vi "Finish.vi"   [LabVIEW 2016]
doc: "This VI is called just before exiting. It is expected to close I/O refnum, save collected data, etc."
uses:
  <vilib>/Rock Robotics/WPI/Utilities/WPI_GetSetVariantRefNum.vi
types:
  T1 = typedef "WPI_MotorControlDeviceRef.ctl" = cluster{"DeviceStatus":errorcluster, "Type":T2, "PWM":cluster{"PWM Channel":T3, "DeadBand":T4}, "CAN":cluster{"Device Number":u8, "SetOutput VI Ref":variant, "GetOutput VI Ref":variant, "Enable VI Ref":variant, "Disable VI Ref":variant, "Data":variant}, "Invert":bool}
  T2 = typedef "WPI_MotorControlType.ctl" = enum16{"PWM", "CAN"}
  T3 = typedef "FPGA_DIOPWMChannel.ctl" = enum8{"PWM 0", "PWM 1", "PWM 2", "PWM 3", "PWM 4", "PWM 5", "PWM 6", "PWM 7", "PWM 8", "PWM 9", "PWM MXP 0", "PWM MXP 1", "PWM MXP 2", "PWM MXP 3", "PWM MXP 4", "PWM MXP 5", "PWM MXP 6", "PWM MXP 7", "PWM MXP 8", "PWM MXP 9", "Invalid"}
  T4 = typedef "WPI_PWMDeadband.ctl" = cluster{"Name":string, "maxPositivePwm":i32, "minPositivePwm":i32, "centerPwm":i32, "maxNegativePwm":i32, "minNegativePwm":i32, "angularRange":u16}
  T5 = typedef "WPI_RelayDevRef.ctl" = cluster{"DevStatus":errorcluster, "Relay Channel":T6, "Relay Direction":T7}
  T6 = typedef "FPGA_DIORelayChannel.ctl" = enum8{"Relay 0", "Relay 1", "Relay 2", "Relay 3", "Invalid"}
  T7 = typedef "WPI_RelayDirection.ctl" = enum16{"Both directions", "Forward only", "Reverse only"}
  T8 = typedef "WPI_JoystickDevRef.ctl" = cluster{"Device":T9}
  T9 = typedef "WPI_JoystickDeviceEnum.ctl" = enum16{"USB 0", "USB 1", "USB 2", "USB 3", "USB 4", "USB 5"}
  T10 = typedef "WPI_RobotDriveDevRef.ctl" = cluster{"DevStatus":errorcluster, "Motors[]":T1[], "Square Inputs":bool, "Max Output":dbl}
  T11 = typedef "WPI_SolenoidDevRef.ctl" = cluster{"DevStatus":errorcluster, "Pneumatics Control Module":u8, "Forward Solenoid Channel":T12, "Reverse Solenoid Channel":T12}
  T12 = typedef "WPI_SolenoidChannel.ctl" = enum8{"Solenoid 0", "Solenoid 1", "Solenoid 2", "Solenoid 3", "Solenoid 4", "Solenoid 5", "Solenoid 6", "Solenoid 7", "Invalid"}
  T13 = typedef "WPI_CompressorDevRef.ctl" = cluster{"DevStatus":errorcluster, "Pneumatics Control Module":u8}
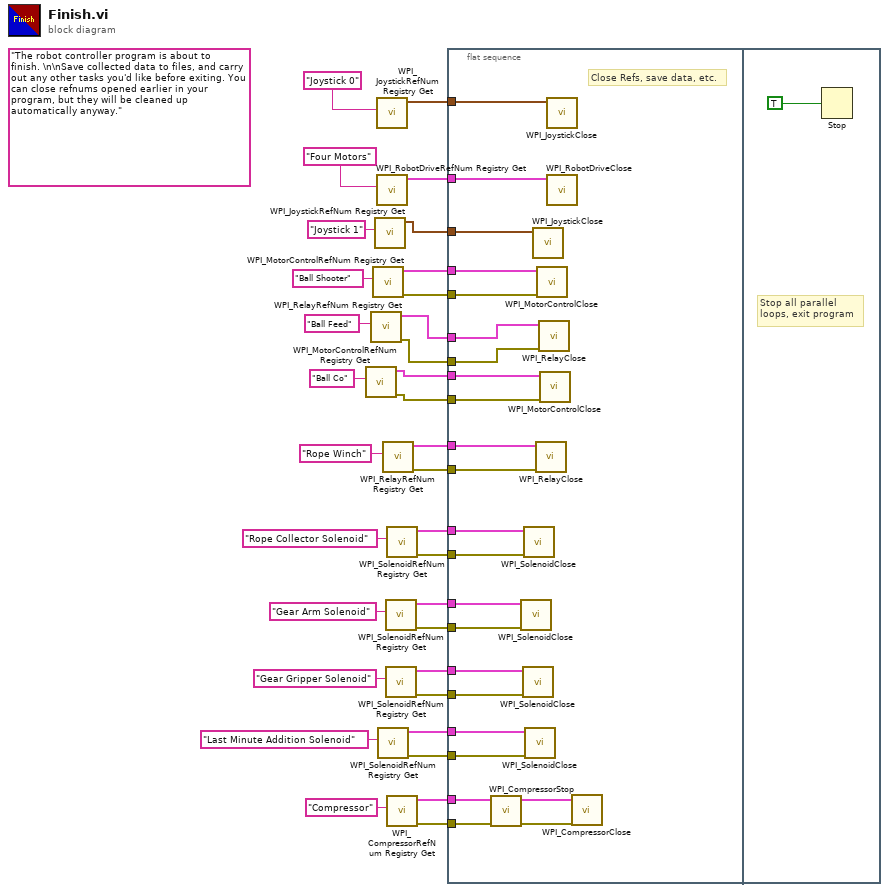
[diagram p0: block diagram]
diagram:
  (unwired) "The robot controller program is about to finish. \n\nSave collected data to files, and carry out any other tasks you'd like before exiting. You can close refnums opened earlier in your program, but they will be cleaned up automatically anyway."
  n1 = call <vilib>:"WPI_MotorControlRefNum Registry Get.vi"("refnum name"="Ball Co") -> ("error out"=w19:errorcluster, "MotorControlDevRef"=w20:T1)  [unwired: 9 in]
  n2 = call <vilib>:"WPI_RelayRefNum Registry Get.vi"("refnum name"="Ball Feed") -> ("error out"=w22:errorcluster, "RelayDevRef"=w23:T5)  [unwired: 9 in]
  n3 = call <vilib>:"WPI_MotorControlRefNum Registry Get.vi"("refnum name"="Ball Shooter") -> ("error out"=w25:errorcluster, "MotorControlDevRef"=w26:T1)  [unwired: 9 in]
  n4 = call <vilib>:"WPI_JoystickRefNum Registry Get.vi"("refnum name"="Joystick 1") -> ("JoystickDevRef"=w28:T8)  [unwired: 1 in, 9 out]
  n5 = call <vilib>:"WPI_JoystickRefNum Registry Get.vi"("refnum name"="Joystick 0") -> ("JoystickDevRef"=w30:T8)  [unwired: 1 in, 9 out]
  n6 = call <vilib>:"WPI_RobotDriveRefNum Registry Get.vi"("refnum name"="Four Motors") -> ("RobotDriveDevRef"=w31:T10)  [unwired: 1 in, 9 out]
  n7 = call <vilib>:"WPI_SolenoidRefNum Registry Get.vi"("refnum name"="Last Minute Addition Solenoid") -> ("error out"=w2:errorcluster, "SolenoidDevRef"=w3:T11)  [unwired: 9 in]
  n8 = call <vilib>:"WPI_RelayRefNum Registry Get.vi"("refnum name"="Rope Winch") -> ("error out"=w16:errorcluster, "RelayDevRef"=w17:T5)  [unwired: 9 in]
  n9 = call <vilib>:"WPI_SolenoidRefNum Registry Get.vi"("refnum name"="Gear Arm Solenoid") -> ("error out"=w8:errorcluster, "SolenoidDevRef"=w9:T11)  [unwired: 9 in]
  n10 = call <vilib>:"WPI_SolenoidRefNum Registry Get.vi"("refnum name"="Gear Gripper Solenoid") -> ("error out"=w5:errorcluster, "SolenoidDevRef"=w6:T11)  [unwired: 9 in]
  n11 = call <vilib>:"WPI_SolenoidRefNum Registry Get.vi"("refnum name"="Rope Collector Solenoid") -> ("error out"=w10:errorcluster, "SolenoidDevRef"=w11:T11)  [unwired: 9 in]
  n12 = call <vilib>:"WPI_CompressorRefNum Registry Get.vi"("refnum name"="Compressor") -> ("error out"=w13:errorcluster, "CompressorDevRef"=w14:T13)  [unwired: 9 in]
  n13 = flat-sequence {
    tunnel: w31 -> [w56]
    tunnel: w30 -> [w55]
    tunnel: w28 -> [w54]
    tunnel: w26 -> [w53]
    tunnel: w25 -> [w52]
    tunnel: w23 -> [w51]
    tunnel: w22 -> [w50]
    tunnel: w20 -> [w49]
    tunnel: w19 -> [w48]
    tunnel: w17 -> [w47]
    tunnel: w16 -> [w46]
    tunnel: w14 -> [w45]
    tunnel: w13 -> [w43]
    tunnel: w11 -> [w41]
    tunnel: w10 -> [w40]
    tunnel: w9 -> [w39]
    tunnel: w8 -> [w38]
    tunnel: w6 -> [w37]
    tunnel: w5 -> [w36]
    tunnel: w3 -> [w35]
    tunnel: w2 -> [w34]
    frame #0 {
      # "Close Refs, save data, etc."
      n14 = call <vilib>:"WPI_CompressorStop.vi"("error in (no error)"=w43, "CompressorDevRef"=w45) -> ("error out"=w42:errorcluster, "CompressorDevRef"=w44:T13)  [unwired: 8 in]
      n15 = call <vilib>:"WPI_SolenoidClose.vi"("error in (no error)"=w38, "SolenoidDevRef"=w39) -> ()  [unwired: 9 in, 1 out]
      n16 = call <vilib>:"WPI_SolenoidClose.vi"("error in (no error)"=w36, "SolenoidDevRef"=w37) -> ()  [unwired: 9 in, 1 out]
      n17 = call <vilib>:"WPI_SolenoidClose.vi"("error in (no error)"=w40, "SolenoidDevRef"=w41) -> ()  [unwired: 9 in, 1 out]
      n18 = call <vilib>:"WPI_SolenoidClose.vi"("error in (no error)"=w34, "SolenoidDevRef"=w35) -> ()  [unwired: 9 in, 1 out]
      n19 = call <vilib>:"WPI_JoystickClose.vi"("JoystickDevRef"=w54) -> ()  [unwired: 11 out]
      n20 = call <vilib>:"WPI_RelayClose.vi"("error in (no error)"=w46, "RelayDevRef"=w47) -> ()  [unwired: 9 in, 1 out]
      n21 = call <vilib>:"WPI_MotorControlClose.vi"("error in"=w52, "MotorControlDevRef"=w53) -> ()  [unwired: 9 in, 1 out]
      n22 = call <vilib>:"WPI_RelayClose.vi"("error in (no error)"=w50, "RelayDevRef"=w51) -> ()  [unwired: 9 in, 1 out]
      n23 = call <vilib>:"WPI_MotorControlClose.vi"("error in"=w48, "MotorControlDevRef"=w49) -> ()  [unwired: 9 in, 1 out]
      n24 = call <vilib>:"WPI_JoystickClose.vi"("JoystickDevRef"=w55) -> ()  [unwired: 11 out]
      n25 = call <vilib>:"WPI_RobotDriveClose.vi"("RobotDriveDevRef"=w56) -> ()  [unwired: 1 in, 10 out]
      n26 = call <vilib>:"WPI_CompressorClose.vi"("error in (no error)"=w42, "CompressorDevRef"=w44) -> ()  [unwired: 9 in, 1 out]
    }
    frame #1 {
      # "Stop all parallel\nloops, exit program"
      n27 = Stop(stop? (T)=TRUE ("Quit")) -> ()
    }
  }
